vi "SAE_stage_control.vi"(6 "error in":errorcluster, 9 "Cluster IN":T1={"Up"=FALSE, "Left"=FALSE, "Right"=FALSE, "Down"=FALSE, "Focus Down"=FALSE, "Focus Up"=FALSE, "X Step Size(um)"=6.860690000000502, "Z step size (um)"=100.0, "Y Step Size(um)"=100.0, "X Position"=0.0, "Y Position"=0.0, "Z Position"=0.0, "Enable x-axis"=FALSE, "Enable y-axis"=FALSE, "Enable z-axis"=FALSE}) -> (0 "error out":errorcluster, 3 "Cluster OUT":T1={"Up"=FALSE, "Left"=FALSE, "Right"=FALSE, "Down"=FALSE, "Focus Down"=FALSE, "Focus Up"=FALSE, "X Step Size(um)"=6.860690000000502, "Z step size (um)"=100.0, "Y Step Size(um)"=100.0, "X Position"=0.0, "Y Position"=0.0, "Z Position"=0.0, "Enable x-axis"=FALSE, "Enable y-axis"=FALSE, "Enable z-axis"=FALSE})   [LabVIEW 2020]
uses:
  typedefs/typedef_stage_control.ctl
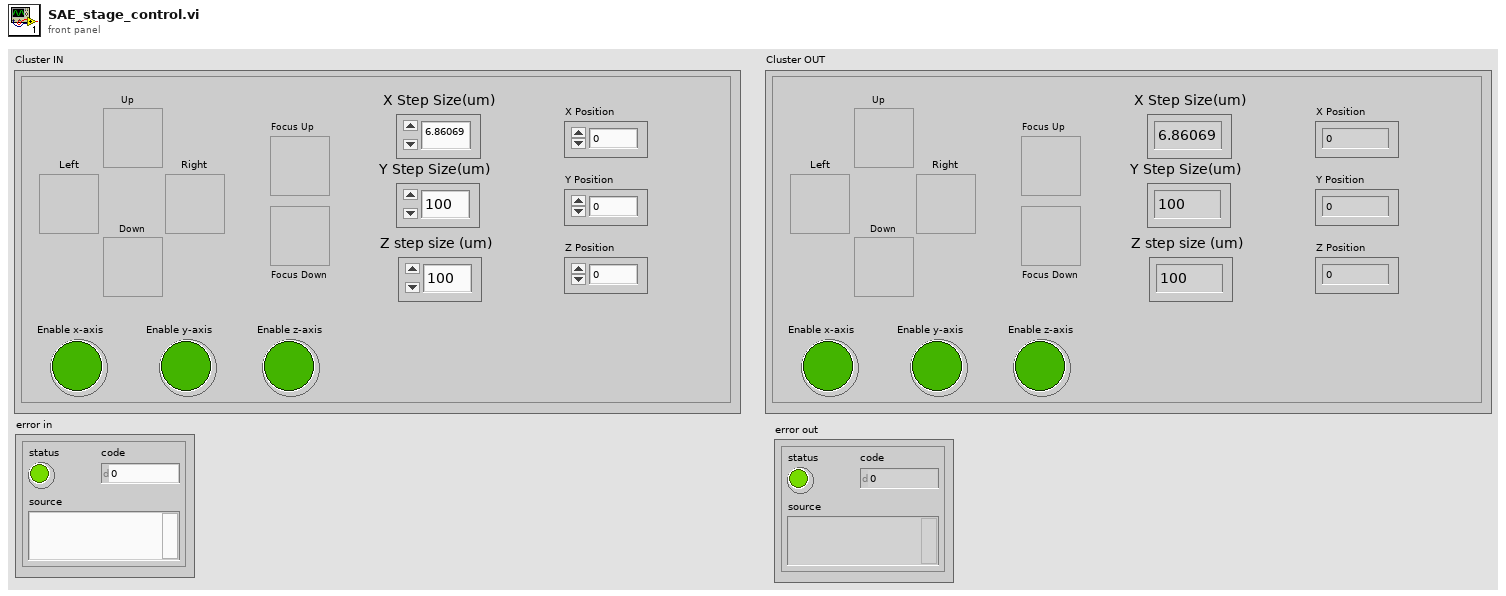
[diagram p1: front panel]
types:
  T1 = typedef "typedef_stage_control.ctl" = cluster{"Up":bool, "Left":bool, "Right":bool, "Down":bool, "Focus Down":bool, "Focus Up":bool, "X Step Size(um)":dbl, "Z step size (um)":dbl, "Y Step Size(um)":dbl, "X Position":dbl, "Y Position":dbl, "Z Position":dbl, "Enable x-axis":bool, "Enable y-axis":bool, "Enable z-axis":bool}
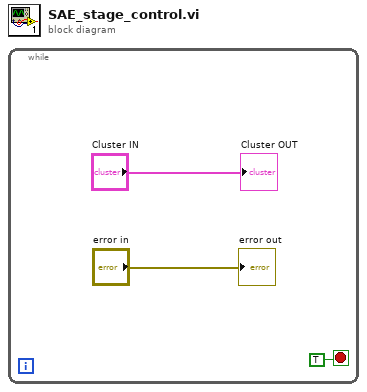
[diagram p0: block diagram]
diagram:
  n1 = while {
    stop <- TRUE stop-if-true
    "Cluster OUT" <- "Cluster IN"
    "error out" <- "error in"
  }
